vi "sine wave.vi"() -> ()   [LabVIEW 2021]
uses:
  <vilib>/express/express analysis/Spectral/Block/exnSpectralBlock spectral measurements peak poly.vi
  <vilib>/express/express analysis/Spectral/Block/exnSpectralBlock spectral measurements peak DDT.vi
  <vilib>/express/express analysis/Spectral/XNode/ExpressSpectralMeasurementsBlockNode.xnode
panel:
  out "?":dynamicdata(graph)
  out "?":dynamicdata(graph)
  out "Waveform Graph with \nhanning":dynamicdata(graph)
  out "Waveform Graph with\n squar window":dynamicdata(graph)
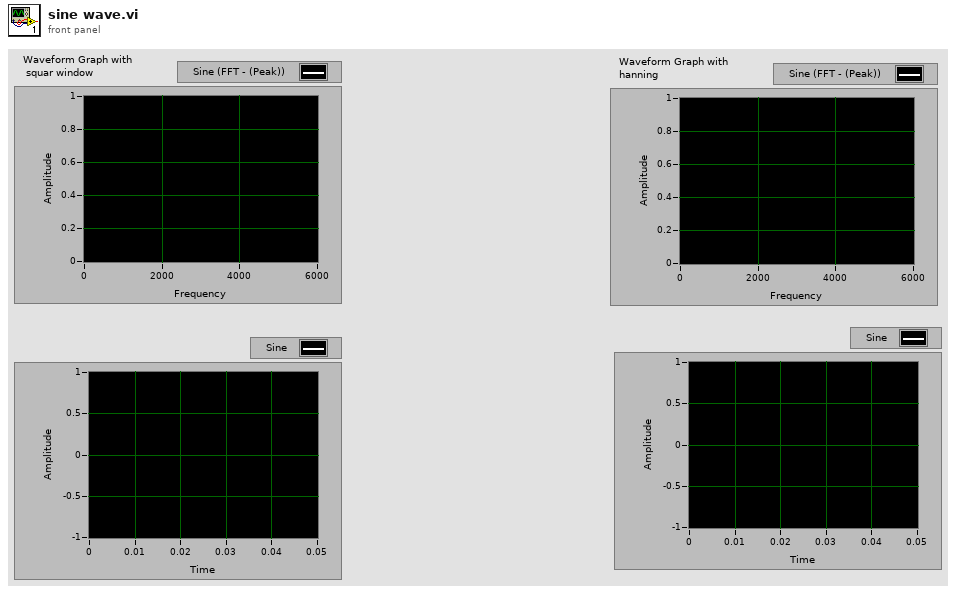
[diagram p1: front panel]
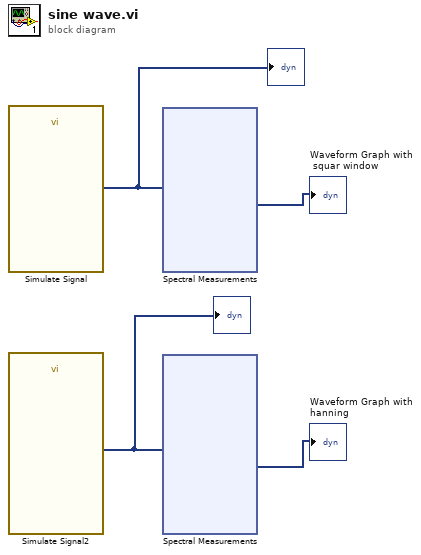
[diagram p0: block diagram]
diagram:
  n1 = call "Simulate Signal"() -> ("Sine"=w2:dynamicdata)  [unwired: 14 in, 1 out]
  "?" <- w2
  n2 = call "Simulate Signal2"() -> ("Sine"=w1:dynamicdata)  [unwired: 14 in, 1 out]
  "?" <- w1
  n3 = xnode "Spectral Measurements"("Signals"=w2) -> ("FFT - (Peak)"=→"Waveform Graph with\n squar window":dynamicdata)  [unwired: 1 in, 2 out]
  n4 = xnode "Spectral Measurements"("Signals"=w1) -> ("FFT - (Peak)"=→"Waveform Graph with \nhanning":dynamicdata)  [unwired: 1 in, 2 out]
